vi "GUI_CH4_Rx.vi"() -> ()   [LabVIEW 2018]
uses:
  Stream/Stream.lvclass
  RxTx/RxTx.lvclass
  Stream/Stream.lvclass/Stream.ctl
panel:
  in  "RxTx.lvclass":refnum<class "RxTx.lvclass">
  in  "Stream.lvclass":refnum<class "Stream.lvclass">
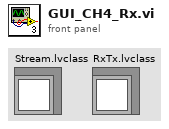
[diagram p1: front panel]
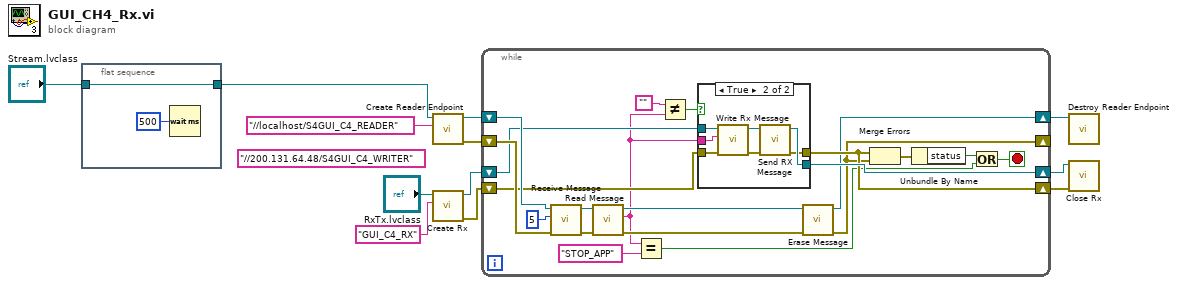
[diagram p0: block diagram]
diagram:
  (unwired) "//200.131.64.48/S4GUI_C4_WRITER" ("witer name")
  n1 = flat-sequence {
    tunnel: "Stream.lvclass" -> [w14]
    tunnel: [w14] -> w1
    frame #0 {
      n2 = Wait (ms)(milliseconds to wait=u32 500) -> ()  [unwired: 1 out]
    }
  }
  n3 = call "Create Reader Endpoint.vi"("reader name"="//localhost/S4GUI_C4_READER", "Stream in"=w1) -> ("error out"=w10:errorcluster, "Stream out"=w11:refnum<class "Stream.lvclass">)  [unwired: 8 in]
  n4 = call "Create Rx.vi"("Reader Name"="GUI_C4_RX", "RxTx in"="RxTx.lvclass") -> ("error out"=w5:errorcluster, "RxTx out"=w6:refnum<class "RxTx.lvclass">)  [unwired: 8 in]
  n5 = while {
    shift-right: [w20] -> _
    shift-left: w10 -> [w34]
    shift-right: [w23] -> w9
    shift-left: w11 -> [w35]
    shift-right: [w27] -> w3
    shift-left: w5 -> [w31]
    shift-right: [w29] -> w4
    shift-left: w6 -> [w30]
    stop <- w17 stop-if-true
    n6 = call "Receive Message.vi"("error in (no error)"=w34, "timeout ms"=5, "Stream in"=w35) -> ("error out"=w32:errorcluster, "Stream out"=w33:refnum<class "Stream.lvclass">)  [unwired: 7 in]
    n7 = call "Read Message.vi"("error in (no error)"=w32, "Stream in"=w33) -> ("error out"=w22:errorcluster, "Message"=w19:string, "Stream out"=w21:refnum<class "Stream.lvclass">)  [unwired: 7 in]
    n8 = Equal?(x=w19, y="STOP_APP" ("reader name")) -> (x = y?=w15:bool)
    n9 = Not Equal?(x="", y=w19) -> (x != y?=w24:bool)
    n10 = case shown="True" w24 {
      tunnel: w31 -> [w36 w42]
      tunnel: w30 -> [w37 w41]
      tunnel: w19 -> [_ w40]
      tunnel: [w37 w39] -> w29
      tunnel: [w36 w38] -> w27
      frame False {
      }
      frame True {
        n11 = call "Write Rx Message.vi"("error in (no error)"=w42, "Rx Message"=w40, "RxTx in"=w41) -> ("error out"=w43:errorcluster, "RxTx out"=w44:refnum<class "RxTx.lvclass">)  [unwired: 7 in]
        n12 = call "Send RX Message.vi"("error in (no error)"=w43, "RxTx in"=w44) -> ("error out"=w38:errorcluster, "RxTx out"=w39:refnum<class "RxTx.lvclass">)  [unwired: 8 in]
      }
    }
    n13 = call "Erase Message.vi"("error in (no error)"=w22, "Stream in"=w21) -> ("error out"=w20:errorcluster, "Stream out"=w23:refnum<class "Stream.lvclass">)  [unwired: 8 in]
    n14 = Merge Errors(w27, w20) -> (w28:errorcluster)
    n15 = Unbundle By Name(w28) -> ("status"=w16:bool)
    n16 = Or(x=w16, y=w15) -> (x .or. y?=w17:bool)
  }
  n17 = call "Destroy Reader Endpoint.vi"("Stream in"=w9) -> ()  [unwired: 9 in, 2 out]
  n18 = call "Close Rx.vi"("error in (no error)"=w3, "RxTx in"=w4) -> ()  [unwired: 8 in, 2 out]
